vi "ReadBacklogFromFile.vi"(8 "error in (no error)":errorcluster, 11 "log dir":path) -> (0 "error out":errorcluster, 3 "backlog messages":T1[](array[typedef]))   [LabVIEW 2017, in "TracePointSynchronizer.lvlib"]
uses:
  <vilib>/addons/InsightCM/Devices/Shared/Common/TracePointSynchronizer/TracePointSynchronizer.lvlib
  <vilib>/addons/InsightCM/MessageBus/Base/controls/Message.ctl
  <vilib>/addons/InsightCM/MessageBus/Base/controls/MessageHeader.ctl
  <vilib>/addons/InsightCM/MessageBus/Base/controls/KeyValuePair.ctl
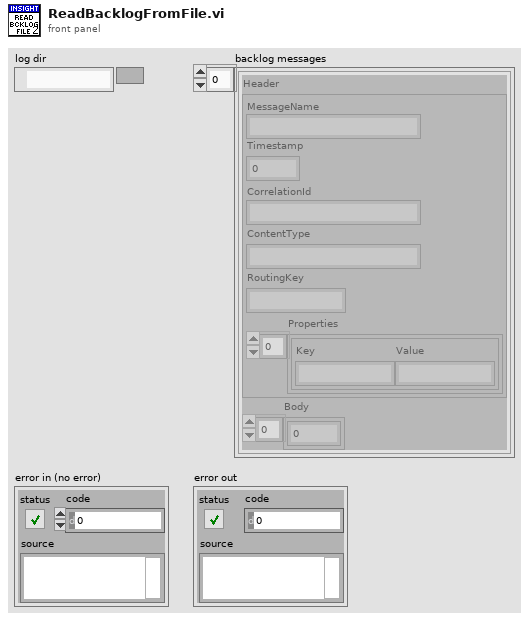
[diagram p1: front panel]
types:
  T1 = typedef "Message.ctl" = cluster{"Header":T2, "Body":u8[]}
  T2 = typedef "MessageHeader.ctl" = cluster{"MessageName":string, "Timestamp":i64, "CorrelationId":string, "ContentType":string, "RoutingKey":string, "Properties":T3[]}
  T3 = typedef "KeyValuePair.ctl" = cluster{"Key":string, "Value":string}
  T4 = enum16{"open", "replace", "create", "open or create", "replace or create", "replace or create with confirmation"}
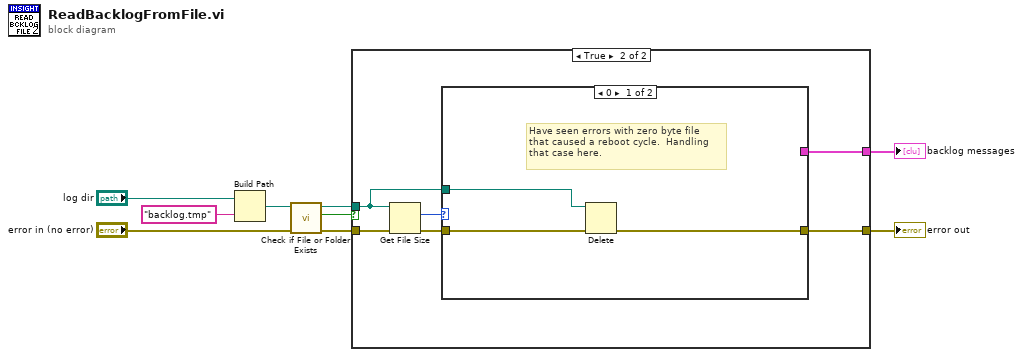
[diagram p0: block diagram]
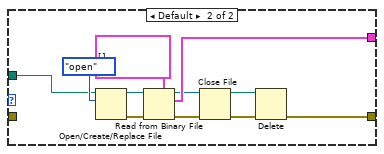
[diagram p3: hidden frame]
diagram:
  n1 = Build Path(base path="log dir", name or relative path="backlog.tmp") -> (appended path=w3:path)
  n2 = call <vilib>:"Check if File or Folder Exists.vi"("error in (no error)"="error in (no error)", "path"=w3) -> ("error out"=w5:errorcluster, "file or folder exists?"=w1:bool, "dup path"=w2:path)  [unwired: 7 in]
  n3 = case shown="True" w1 {
    tunnel: [_ w16] -> w7
    tunnel: [w10 w15] -> w6
    tunnel: w5 -> [w10 w14]
    tunnel: w2 -> [_ w11]
    frame False {
    }
    frame True {
      n4 = Get File Size(file=w11, error in=w14) -> (size (in bytes)=w13:i64, 0:w12:errorcluster)  [unwired: 1 out]
      n5 = case shown="0" w13 {
        tunnel: [_ w27] -> w16
        tunnel: [w17 w21] -> w15
        tunnel: w12 -> [w18 _]
        tunnel: w11 -> [w19 w20]
        frame 0 {
          # "Have seen errors with zero byte file\nthat caused a reboot cycle.  Handling\nthat case here."
          n6 = Delete(path (use dialog)=w19, error in=w18) -> (error out=w17:errorcluster)  [unwired: 3 in, 2 out]
        }
        frame Default {
          n7 = Open/Create/Replace File(file path (use dialog)=w20, operation (0:open)=T4."open") -> (refnum out=w29:refnum<file>, error out=w26:errorcluster)  [unwired: 4 in, 1 out]
          n8 = Read from Binary File(5:T1[] [] ("backlog messages"), 8:w26, 11:w29) -> (0:w24:errorcluster, 2:w27:T1[], 3:w25:refnum<file>)  [unwired: 3 in, 1 out]
          n9 = Close File(refnum=w25, error in=w24) -> (path=w22:path, error out=w23:errorcluster)
          n10 = Delete(path (use dialog)=w22, error in=w23) -> (error out=w21:errorcluster)  [unwired: 3 in, 2 out]
        }
      }
    }
  }
  "error out" <- w6
  "backlog messages" <- w7
